vi "LookAheadPoint.vi"(6 "Reset":bool, 8 "Robot":cluster{"x":dbl, "y":dbl}, 9 "Spacing":dbl, 10 "LookAhead":dbl, 11 "Path":cluster{"x":dbl, "y":dbl}[](array[cluster])) -> (2 "LookaheadIndex":i32, 3 "Point":cluster{"x":dbl, "y":dbl})   [LabVIEW 2017]
doc: "Finds the lookahead point given a path and the current location of the robot."
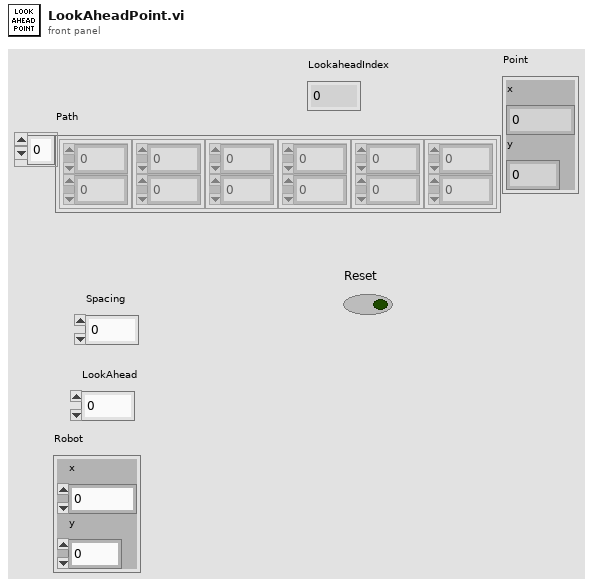
[diagram p1: front panel]
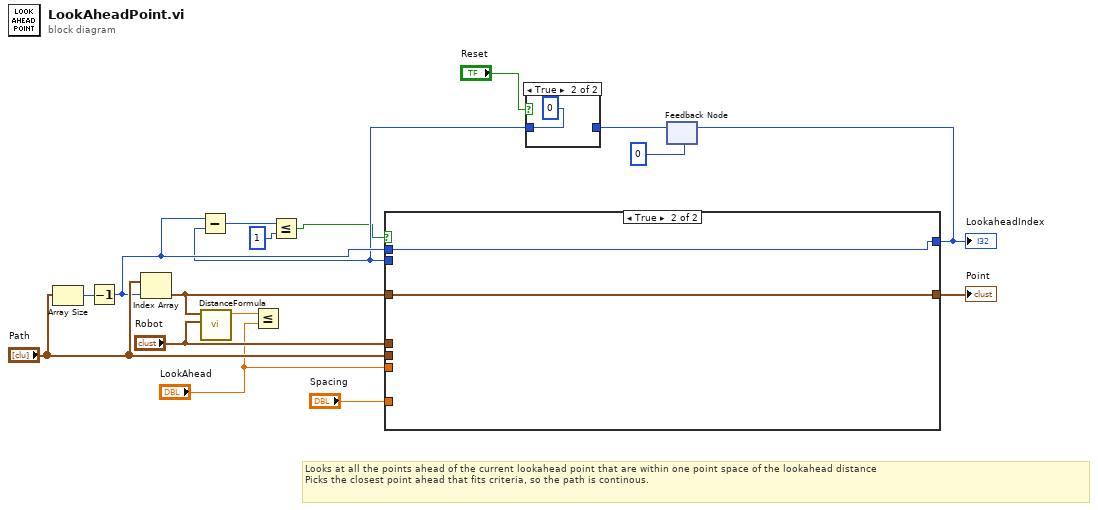
[diagram p0: block diagram]
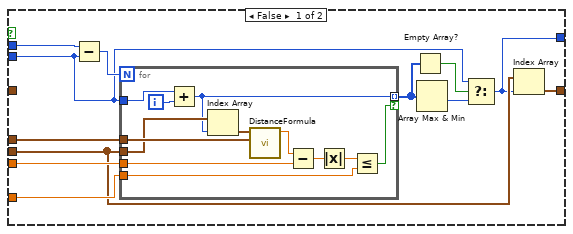
[diagram p3: hidden frame]
diagram:
  # "Looks at all the points ahead of the current lookahead point that are within one point space of the lookahead distance\nPicks the closest point ahead that fits criteria, so the path is continous."
  n1 = Array Size(array="Path") -> (size(s)=w16:i32)
  n2 = Decrement(x=w16) -> (x-1=w8:i32)
  n3 = Index Array(array="Path", index=w8) -> (element=w12:cluster{"x":dbl, "y":dbl})
  n4 = call "DistanceFormula.vi"("Point 2"="Robot", "Point 1"=w12) -> ("Distance"=w10:dbl)  [unwired: 9 in]
  n5 = Less Or Equal?(x=w10, y="LookAhead") -> ()  [unwired: 1 out]
  n6 = feedback #1(0) -> (w3:i32)
  n7 = case shown="True" "Reset" {
    tunnel: w3 -> [w18 _]
    tunnel: [w18 0] -> w4
    frame False {
    }
    frame True {
    }
  }
  n8 = Subtract(x=w8, y=w4) -> (x-y=w7:i32)
  n9 = Less Or Equal?(x=w7, y=1) -> (x <= y?=w1:bool)
  n10 = case shown="True" w1 {
    tunnel: "LookAhead" -> [w31 _]
    tunnel: [w30 w45] -> w17
    tunnel: "Path" -> [w25 _]
    tunnel: "Robot" -> [w29 _]
    tunnel: [w20 w44] -> w2
    tunnel: w12 -> [_ w45]
    tunnel: w8 -> [w28 w44]
    tunnel: "Spacing" -> [w26 _]
    tunnel: w4 -> [w21 _]
    frame False {
      n11 = Subtract(x=w28, y=w21) -> (x-y=w27:i32)
      n12 = for {
        N: w27 -> [_]
        tunnel: w25 -> [w40]
        tunnel: w29 -> [w43]
        tunnel: w31 -> [w42]
        tunnel: w21 -> [w38]
        tunnel: w26 -> [w35]
        tunnel: [w34] -> w24 mode=indexing if=w33
        i -> [w39]
        n13 = Add(x=w38, y=w39) -> (x+y=w34:i32)
        n14 = Index Array(array=w40, index=w34) -> (element=w37:cluster{"x":dbl, "y":dbl})
        n15 = call "DistanceFormula.vi"("Point 2"=w43, "Point 1"=w37) -> ("Distance"=w32:dbl)  [unwired: 9 in]
        n16 = Subtract(x=w32, y=w42) -> (x-y=w41:dbl)
        n17 = Absolute Value(x=w41) -> (abs(x)=w36:dbl)
        n18 = Less Or Equal?(x=w36, y=w35) -> (x <= y?=w33:bool)
      }
      n19 = Empty Array?(array=w24) -> (empty?=w23:bool)
      n20 = Array Max & Min(array=w24) -> (min value=w22:i32)  [unwired: 3 out]
      n21 = Select(t=w21, s=w23, f=w22) -> (s? t:f=w20:i32)
      n22 = Index Array(array=w25, index=w20) -> (element=w30:cluster{"x":dbl, "y":dbl})
    }
    frame True {
    }
  }
  "Point" <- w17
  "LookaheadIndex" <- w2
  n23 = feedback-in #1(w2) -> ()
